vi "LinearSolve.vi"(2 "Line 2":cluster{"M":dbl, "B":dbl}, 3 "Line 1":cluster{"M":dbl, "B":dbl}) -> (0 "Y":dbl, 1 "X":dbl)   [LabVIEW 2011]
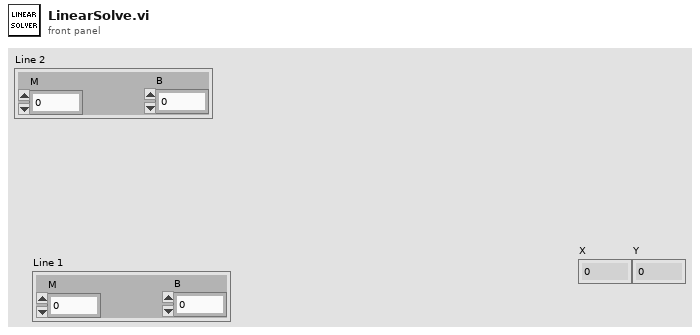
[diagram p1: front panel]
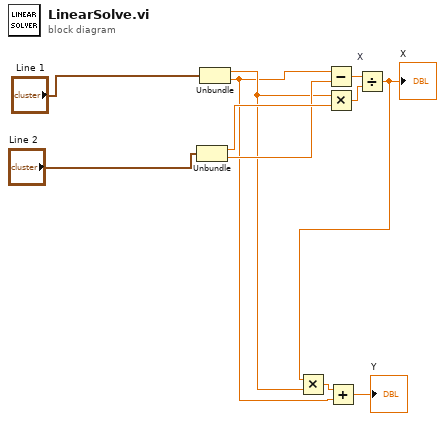
[diagram p0: block diagram]
diagram:
  n1 = Unbundle("Line 2") -> ("M"=w9:dbl, "B"=w8:dbl)
  n2 = Unbundle("Line 1") -> ("M"=w3:dbl, "B"=w2:dbl)
  n3 = Subtract(x=w2, y=w8) -> (x-y=w11:dbl)
  n4 = Multiply(x=w3, y=w9) -> (x*y=w10:dbl)
  n5 = Divide "X"(x=w11, y=w10) -> (x/y=w4:dbl)
  "X" <- w4
  n6 = Multiply(x=w4, y=w3) -> (x*y=w5:dbl)
  n7 = Add(x=w5, y=w2) -> (x+y=→"Y":dbl)
